vi "Recorded Values.vi"(11 "Path":path) -> (1 "Recorded Char":T3, 2 "Recorded Prop":T2, 3 "Fabrication Prop":T1)   [LabVIEW 2012]
uses:
  <vilib>/Utility/file.llb/Read From Spreadsheet File (string).vi
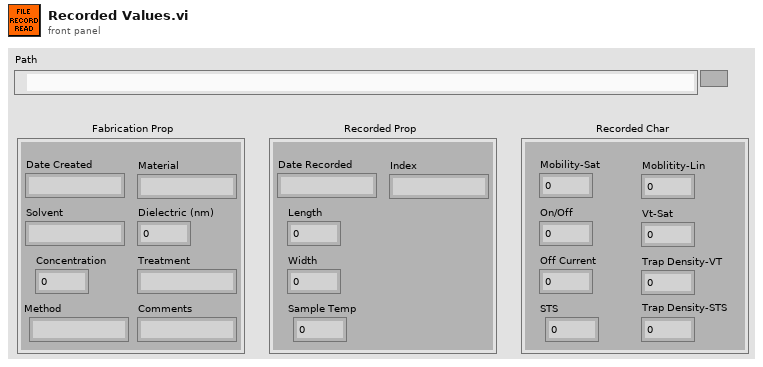
[diagram p1: front panel]
types:
  T1 = cluster{"Date Created":string, "Material":string, "Solvent":string, "Concentration":dbl, "Method":string, "Dielectric (nm)":dbl, "Treatment":string, "Comments":string}
  T2 = cluster{"Date Recorded":string, "Index":string, "Length":dbl, "Width":dbl, "Sample Temp":dbl}
  T3 = cluster{"Mobility-Sat":dbl, "Moblitity-Lin":dbl, "On/Off":dbl, "Off Current":dbl, "Vt-Sat":dbl, "STS":dbl, "Trap Density-VT":dbl, "Trap Density-STS":dbl}
  T4 = cluster{"String":string, "String":string, "String":string, dbl, "String":string, dbl, "String":string, "String":string}
  T5 = cluster{"String":string, "String":string, dbl, dbl, dbl}
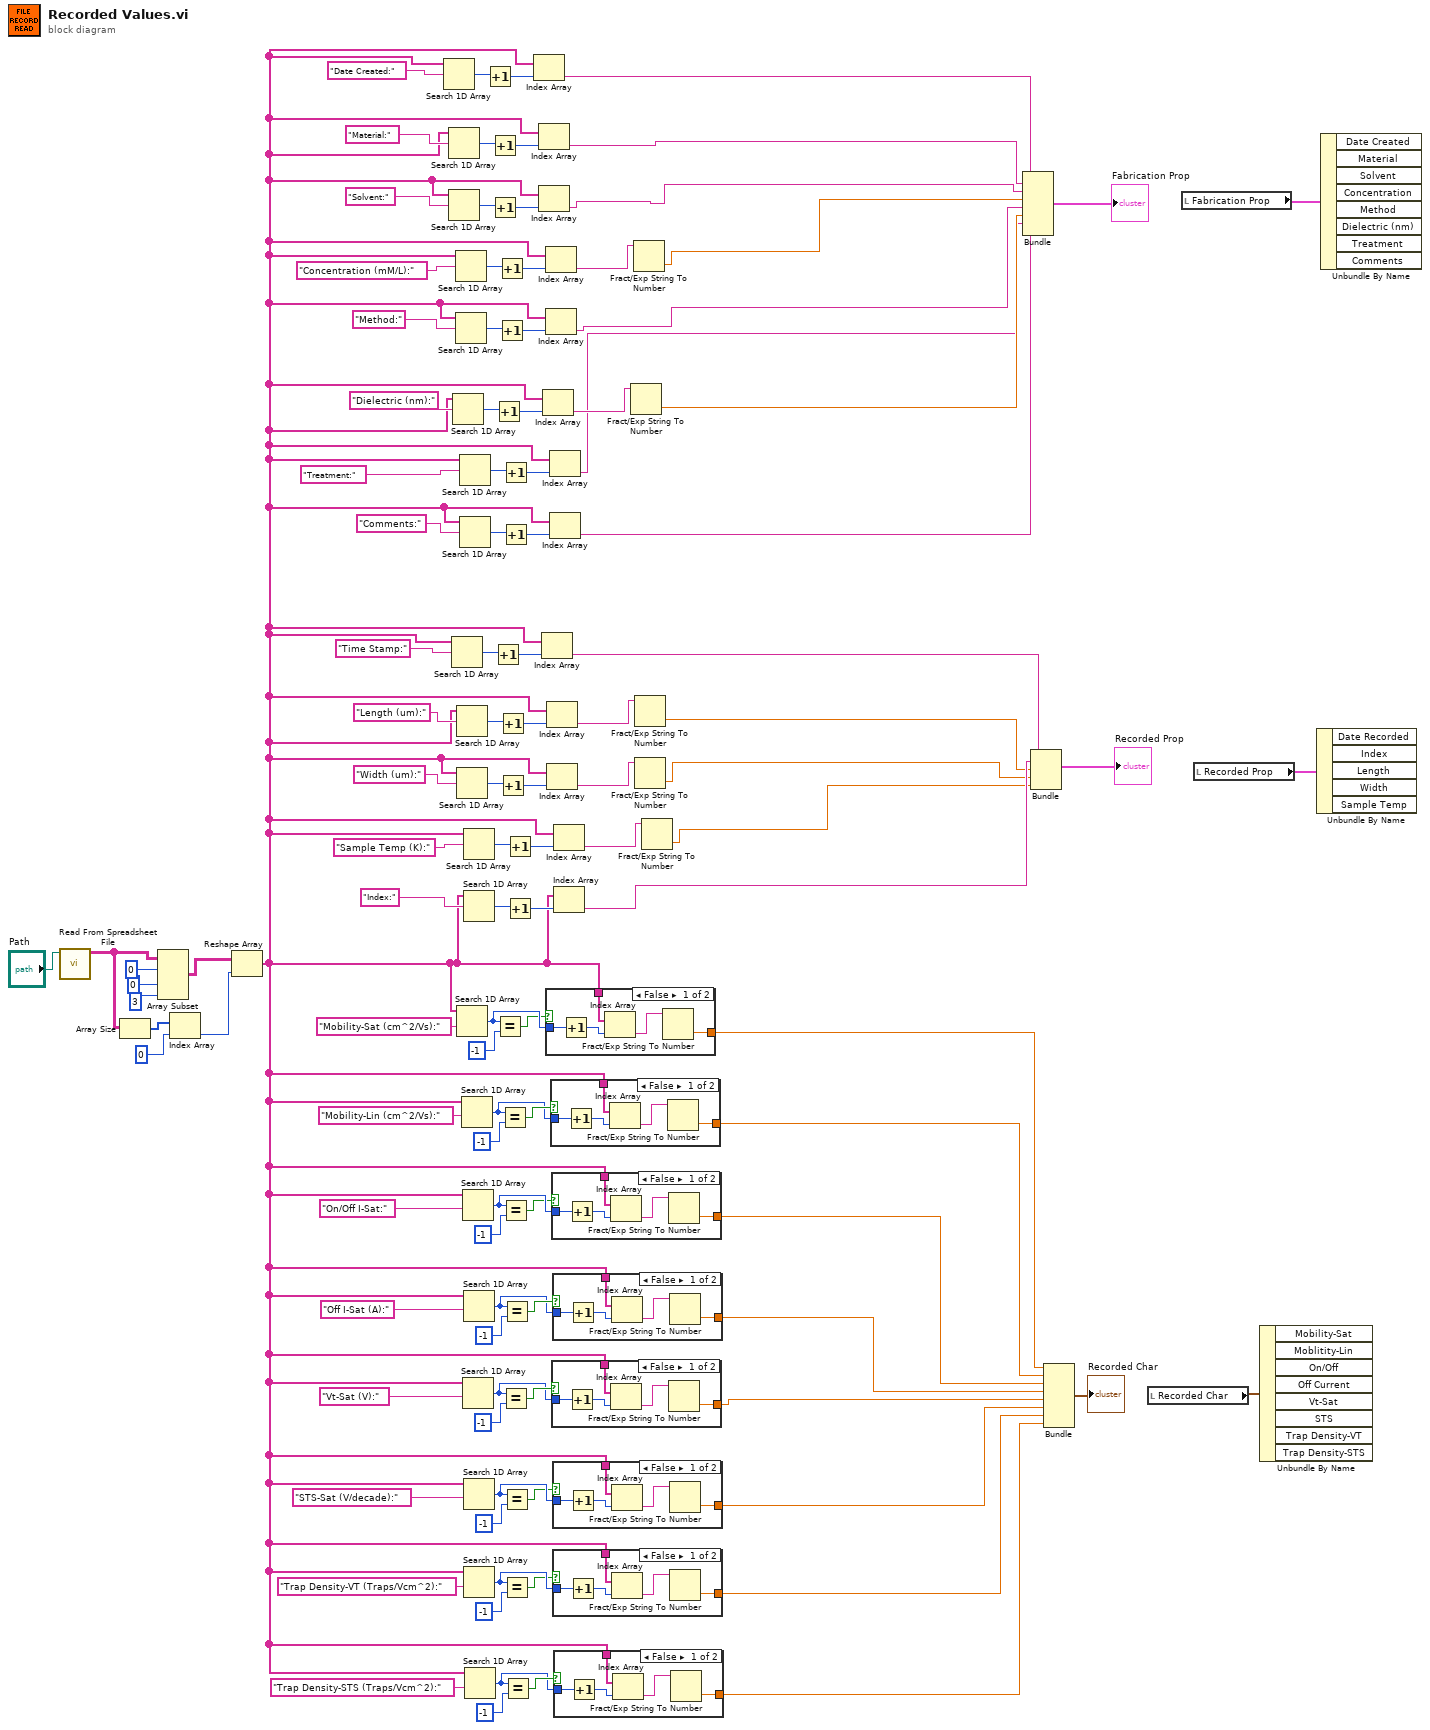
[diagram p0: block diagram]
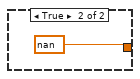
[diagram p2: hidden frame]
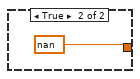
[diagram p3: hidden frame]
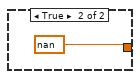
[diagram p4: hidden frame]
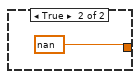
[diagram p5: hidden frame]
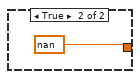
[diagram p6: hidden frame]
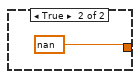
[diagram p7: hidden frame]
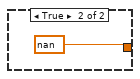
[diagram p8: hidden frame]
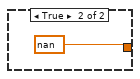
[diagram p9: hidden frame]
diagram:
  n1 = call-poly <vilib>:"Read From Spreadsheet File.vi"("file path (dialog if empty)"="Path") -> ("all rows"=w108:string[][])  [unwired: 6 in, 4 out]
  n2 = Array Size(array=w108) -> (size(s)=w107:i32[])
  n3 = Array Subset(array=w108, index (row)=0, index (col)=0, length (col)=3) -> (w109:string[][])  [unwired: 1 in]
  n4 = Index Array(array=w107, index=0) -> (element=w105:i32)
  n5 = Reshape Array(w109, w105) -> (w11:string[])
  n6 = Search 1D Array(1D array=w11, element="Date Created:") -> (index of element=w29:i32)  [unwired: 1 in]
  n7 = Search 1D Array(1D array=w11, element="Material:") -> (index of element=w23:i32)  [unwired: 1 in]
  n8 = Search 1D Array(1D array=w11, element="Solvent:") -> (index of element=w26:i32)  [unwired: 1 in]
  n9 = Search 1D Array(1D array=w11, element="Time Stamp:") -> (index of element=w53:i32)  [unwired: 1 in]
  n10 = Search 1D Array(1D array=w11, element="Dielectric (nm):") -> (index of element=w20:i32)  [unwired: 1 in]
  n11 = Search 1D Array(1D array=w11, element="Concentration (mM/L):") -> (index of element=w36:i32)  [unwired: 1 in]
  n12 = Search 1D Array(1D array=w11, element="Method:") -> (index of element=w32:i32)  [unwired: 1 in]
  n13 = Search 1D Array(1D array=w11, element="Length (um):") -> (index of element=w61:i32)  [unwired: 1 in]
  n14 = Search 1D Array(1D array=w11, element="Width (um):") -> (index of element=w57:i32)  [unwired: 1 in]
  n15 = Search 1D Array(1D array=w11, element="Mobility-Sat (cm^2/Vs):") -> (index of element=w104:i32)  [unwired: 1 in]
  n16 = Search 1D Array(1D array=w11, element="Treatment:") -> (index of element=w13:i32)  [unwired: 1 in]
  n17 = Search 1D Array(1D array=w11, element="Comments:") -> (index of element=w16:i32)  [unwired: 1 in]
  n18 = Search 1D Array(1D array=w11, element="Mobility-Lin (cm^2/Vs):") -> (index of element=w96:i32)  [unwired: 1 in]
  n19 = Search 1D Array(1D array=w11, element="On/Off I-Sat:") -> (index of element=w93:i32)  [unwired: 1 in]
  n20 = Search 1D Array(1D array=w11, element="Vt-Sat (V):") -> (index of element=w78:i32)  [unwired: 1 in]
  n21 = Search 1D Array(1D array=w11, element="Sample Temp (K):") -> (index of element=w46:i32)  [unwired: 1 in]
  n22 = Search 1D Array(1D array=w11, element="Index:") -> (index of element=w50:i32)  [unwired: 1 in]
  n23 = Search 1D Array(1D array=w11, element="Off I-Sat (A):") -> (index of element=w86:i32)  [unwired: 1 in]
  n24 = Search 1D Array(1D array=w11, element="STS-Sat (V/decade):") -> (index of element=w85:i32)  [unwired: 1 in]
  n25 = Search 1D Array(1D array=w11, element="Trap Density-VT (Traps/Vcm^2):") -> (index of element=w77:i32)  [unwired: 1 in]
  n26 = Search 1D Array(1D array=w11, element="Trap Density-STS (Traps/Vcm^2):") -> (index of element=w70:i32)  [unwired: 1 in]
  n27 = Increment(x=w29) -> (x+1=w28:i32)
  n28 = Increment(x=w23) -> (x+1=w24:i32)
  n29 = Increment(x=w26) -> (x+1=w25:i32)
  n30 = Increment(x=w53) -> (x+1=w54:i32)
  n31 = Increment(x=w20) -> (x+1=w21:i32)
  n32 = Equal?(x=w104, y=-1) -> (x = y?=w103:bool)
  n33 = Increment(x=w36) -> (x+1=w35:i32)
  n34 = Increment(x=w32) -> (x+1=w33:i32)
  n35 = Increment(x=w61) -> (x+1=w60:i32)
  n36 = Increment(x=w57) -> (x+1=w58:i32)
  n37 = Equal?(x=w96, y=-1) -> (x = y?=w97:bool)
  n38 = Increment(x=w13) -> (x+1=w14:i32)
  n39 = Increment(x=w16) -> (x+1=w15:i32)
  n40 = Equal?(x=w93, y=-1) -> (x = y?=w92:bool)
  n41 = Equal?(x=w78, y=-1) -> (x = y?=w79:bool)
  n42 = Equal?(x=w86, y=-1) -> (x = y?=w87:bool)
  n43 = Equal?(x=w85, y=-1) -> (x = y?=w84:bool)
  n44 = Equal?(x=w77, y=-1) -> (x = y?=w76:bool)
  n45 = Equal?(x=w70, y=-1) -> (x = y?=w71:bool)
  n46 = Increment(x=w46) -> (x+1=w47:i32)
  n47 = Increment(x=w50) -> (x+1=w49:i32)
  n48 = Index Array(array=w11, index=w28) -> (element=w40:string)
  n49 = Index Array(array=w11, index=w24) -> (element=w10:string)
  n50 = Index Array(array=w11, index=w25) -> (element=w9:string)
  n51 = Index Array(array=w11, index=w54) -> (element=w42:string)
  n52 = Index Array(array=w11, index=w21) -> (element=w18:string)
  n53 = Index Array(array=w11, index=w35) -> (element=w34:string)
  n54 = Index Array(array=w11, index=w33) -> (element=w8:string)
  n55 = case shown="False" w103 {
    tunnel: w104 -> [w117 _]
    tunnel: w11 -> [w116 _]
    tunnel: [w114 nan] -> w95
    frame False {
      n56 = Increment(x=w117) -> (x+1=w118:i32)
      n57 = Index Array(array=w116, index=w118) -> (element=w115:string)
      n58 = Fract/Exp String To Number(string=w115) -> (number=w114:dbl)  [unwired: 3 in, 1 out]
    }
    frame True {
    }
  }
  n59 = Index Array(array=w11, index=w60) -> (element=w59:string)
  n60 = Index Array(array=w11, index=w58) -> (element=w55:string)
  n61 = Index Array(array=w11, index=w14) -> (element=w6:string)
  n62 = Index Array(array=w11, index=w15) -> (element=w5:string)
  n63 = case shown="False" w97 {
    tunnel: w96 -> [w123 _]
    tunnel: w11 -> [w122 _]
    tunnel: [w120 nan] -> w94
    frame False {
      n64 = Increment(x=w123) -> (x+1=w124:i32)
      n65 = Index Array(array=w122, index=w124) -> (element=w121:string)
      n66 = Fract/Exp String To Number(string=w121) -> (number=w120:dbl)  [unwired: 3 in, 1 out]
    }
    frame True {
    }
  }
  n67 = case shown="False" w92 {
    tunnel: w93 -> [w129 _]
    tunnel: w11 -> [w128 _]
    tunnel: [w126 nan] -> w69
    frame False {
      n68 = Increment(x=w129) -> (x+1=w130:i32)
      n69 = Index Array(array=w128, index=w130) -> (element=w127:string)
      n70 = Fract/Exp String To Number(string=w127) -> (number=w126:dbl)  [unwired: 3 in, 1 out]
    }
    frame True {
    }
  }
  n71 = case shown="False" w79 {
    tunnel: w78 -> [w135 _]
    tunnel: w11 -> [w134 _]
    tunnel: [w132 nan] -> w67
    frame False {
      n72 = Increment(x=w135) -> (x+1=w136:i32)
      n73 = Index Array(array=w134, index=w136) -> (element=w133:string)
      n74 = Fract/Exp String To Number(string=w133) -> (number=w132:dbl)  [unwired: 3 in, 1 out]
    }
    frame True {
    }
  }
  n75 = case shown="False" w87 {
    tunnel: w86 -> [w141 _]
    tunnel: w11 -> [w140 _]
    tunnel: [w138 nan] -> w68
    frame False {
      n76 = Increment(x=w141) -> (x+1=w142:i32)
      n77 = Index Array(array=w140, index=w142) -> (element=w139:string)
      n78 = Fract/Exp String To Number(string=w139) -> (number=w138:dbl)  [unwired: 3 in, 1 out]
    }
    frame True {
    }
  }
  n79 = case shown="False" w84 {
    tunnel: w85 -> [w147 _]
    tunnel: w11 -> [w146 _]
    tunnel: [w144 nan] -> w66
    frame False {
      n80 = Increment(x=w147) -> (x+1=w148:i32)
      n81 = Index Array(array=w146, index=w148) -> (element=w145:string)
      n82 = Fract/Exp String To Number(string=w145) -> (number=w144:dbl)  [unwired: 3 in, 1 out]
    }
    frame True {
    }
  }
  n83 = case shown="False" w76 {
    tunnel: w77 -> [w153 _]
    tunnel: w11 -> [w152 _]
    tunnel: [w150 nan] -> w65
    frame False {
      n84 = Increment(x=w153) -> (x+1=w154:i32)
      n85 = Index Array(array=w152, index=w154) -> (element=w151:string)
      n86 = Fract/Exp String To Number(string=w151) -> (number=w150:dbl)  [unwired: 3 in, 1 out]
    }
    frame True {
    }
  }
  n87 = Index Array(array=w11, index=w47) -> (element=w48:string)
  n88 = Index Array(array=w11, index=w49) -> (element=w4:string)
  n89 = case shown="False" w71 {
    tunnel: w70 -> [w159 _]
    tunnel: w11 -> [w158 _]
    tunnel: [w156 nan] -> w64
    frame False {
      n90 = Increment(x=w159) -> (x+1=w160:i32)
      n91 = Index Array(array=w158, index=w160) -> (element=w157:string)
      n92 = Fract/Exp String To Number(string=w157) -> (number=w156:dbl)  [unwired: 3 in, 1 out]
    }
    frame True {
    }
  }
  n93 = Fract/Exp String To Number(string=w18) -> (number=w7:dbl)  [unwired: 3 in, 1 out]
  n94 = Fract/Exp String To Number(string=w34) -> (number=w41:dbl)  [unwired: 3 in, 1 out]
  n95 = Fract/Exp String To Number(string=w59) -> (number=w3:dbl)  [unwired: 3 in, 1 out]
  n96 = Fract/Exp String To Number(string=w55) -> (number=w2:dbl)  [unwired: 3 in, 1 out]
  n97 = Fract/Exp String To Number(string=w48) -> (number=w1:dbl)  [unwired: 3 in, 1 out]
  n98 = Bundle("String"=w40, "String"=w10, "String"=w9, w41, "String"=w8, w7, "String"=w6, "String"=w5) -> (→"Fabrication Prop":T4)  [unwired: 1 in]
  n99 = Bundle("String"=w42, "String"=w4, w3, w2, w1) -> (→"Recorded Prop":T5)  [unwired: 1 in]
  n100 = Bundle(w95, w94, w69, w68, w67, w66, w65, w64) -> (→"Recorded Char":cluster{dbl, dbl, dbl, dbl, dbl, dbl, dbl, dbl})  [unwired: 1 in]
  n101 = local read "Recorded Char"() -> (w63:T3)
  n102 = local read "Fabrication Prop"() -> (w38:T1)
  n103 = local read "Recorded Prop"() -> (w44:T2)
  n104 = Unbundle By Name(w63) -> ()  [unwired: 8 out]
  n105 = Unbundle By Name(w44) -> ()  [unwired: 5 out]
  n106 = Unbundle By Name(w38) -> ()  [unwired: 8 out]
